vi "createTopicRefClusterConstant.vi"(8 "error in (no error)":errorcluster, 11 "OpenConnectionInstance in":refnum<class "OpenConnectionInstance.lvclass">) -> (0 "error out":errorcluster, 3 "OpenConnectionInstance out":refnum<class "OpenConnectionInstance.lvclass">)   [LabVIEW 2012, in "OpenConnectionInstance.lvclass"]
uses:
  OpenConnectionInstance.lvclass
  PolymorphicInstance/PolymorphicInstance.lvclass/PolymorphicInstance.ctl
  OpenConnectionInstance.lvclass/OpenConnectionInstance.ctl
  PolymorphicInstance/PolymorphicInstance.lvclass
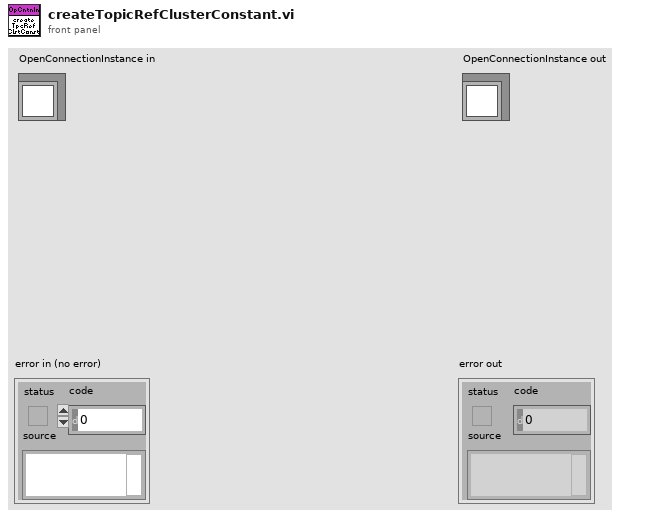
[diagram p1: front panel]
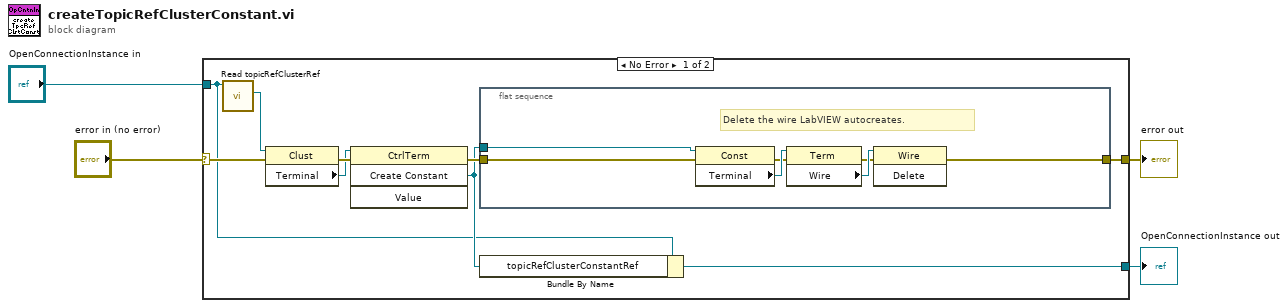
[diagram p0: block diagram]
diagram:
  n1 = case shown="No Error" "error in (no error)" {
    selector: "error in (no error)" -> [w9 w22]
    tunnel: [w8 w22] -> w3
    tunnel: [w5 w21] -> w1
    tunnel: "OpenConnectionInstance in" -> [w6 w21]
    frame No Error {
      n2 = call "Read topicRefClusterRef.vi"("PolymorphicInstance in"=w6) -> ("topicRefClusterRef"=w10:refnum<vi>)  [unwired: 8 in, 2 out]
      n3 = property class="Clust"(reference=w10, error in=w9) -> (error out=w13:errorcluster, "Terminal"=w12:refnum<vi>)  [unwired: 1 out]
      n4 = invoke class="CtrlTerm" method="Create Constant"(reference=w12, error in=w13) -> (error out=w11:errorcluster, "Create Constant"=w7:refnum<vi>)  [unwired: 2 in, 2 out]
      n5 = flat-sequence {
        tunnel: w11 -> [w20]
        tunnel: [w15] -> w8
        tunnel: w7 -> [w14]
        frame #0 {
          # "Delete the wire LabVIEW autocreates."
          n6 = property class="Const"(reference=w14, error in=w20) -> (error out=w17:errorcluster, "Terminal"=w19:refnum<vi>)  [unwired: 1 out]
          n7 = property class="Term"(reference=w19, error in=w17) -> (error out=w16:errorcluster, "Wire"=w18:refnum<vi>)  [unwired: 1 out]
          n8 = invoke class="Wire" method="Delete"(reference=w18, error in=w16) -> (error out=w15:errorcluster)  [unwired: 1 in, 2 out]
        }
      }
      n9 = Bundle By Name(cluster=w6, "topicRefClusterConstantRef"=w7) -> (w5:refnum<class "OpenConnectionInstance.lvclass">)
    }
    frame Error {
    }
  }
  "error out" <- w3
  "OpenConnectionInstance out" <- w1
